vi "07-get-and_display_image.vi"() -> ()   [LabVIEW 2018, in "LV-0mq-Julia_roundtrip-lib.lvlib" / "LV2Julia_examples.lvlib"]
uses:
  LV2Julia_examples.lvlib
  LV2Julia_core/VIs/Server or client state.ctl
  LV2Julia_core/VIs/Commands.ctl
  c965f866-6df0-488f-ad0f-a92a8fae8aa7.vi
  f9264f0d-2c2d-4a22-a0da-9e005a3dfb77.vi
  c965f866-6df0-488f-ad0f-a92a8fae8aa7.vi/5d8143e1-f3ce-48d4-8562-fd4bfbe71124.vi
  f9264f0d-2c2d-4a22-a0da-9e005a3dfb77.vi/0c0e5131-77ab-4bc9-85bf-e376b45f74d3.vi
  c965f866-6df0-488f-ad0f-a92a8fae8aa7.vi/5d8143e1-f3ce-48d4-8562-fd4bfbe71124.vi/85423a51-09b0-429e-94d3-16956556064d.vi
  c965f866-6df0-488f-ad0f-a92a8fae8aa7.vi/5d8143e1-f3ce-48d4-8562-fd4bfbe71124.vi/311e7394-f85c-40bd-9389-6729e46b6738.vi
  c965f866-6df0-488f-ad0f-a92a8fae8aa7.vi/5d8143e1-f3ce-48d4-8562-fd4bfbe71124.vi/bf3cff3a-5cd2-4a77-8ee0-2dd55a1dd824.vi
  f9264f0d-2c2d-4a22-a0da-9e005a3dfb77.vi/0c0e5131-77ab-4bc9-85bf-e376b45f74d3.vi/ed46709f-38a3-410e-bde8-057d058233aa.vi
  f9264f0d-2c2d-4a22-a0da-9e005a3dfb77.vi/0c0e5131-77ab-4bc9-85bf-e376b45f74d3.vi/e79dc27b-6cb8-4aa6-a1cf-490a5ee80ef7.vi
  f9264f0d-2c2d-4a22-a0da-9e005a3dfb77.vi/0c0e5131-77ab-4bc9-85bf-e376b45f74d3.vi/d9315110-f036-4f78-83c6-5fac338d98fa.vi
  LV2Julia_core/VIs/check ID validity.vi
  LV2Julia_core/VIs/bindata_descr to JSON.vi
  LV2Julia_core/VIs/check cluster field names.vi
  LV2Julia_core/VIs/concat JSON.vi
  LV2Julia_core/VIs/build request.vi
  LV2Julia_core/VIs/Parse server response.vi
  LV2Julia_core/VIs/log jl exceptions.vi
  LV2Julia_core/VIs/jl-scripts path.vi
  LV2Julia_core/LV2Julia_core.lvlib
panel:
  out "img_type":string
  out "picture":picture
  in  "select image":u16(ring)
  out "short error info":string
  in  "next":bool
  out "current error":errorcluster
  out "final error":errorcluster
  in  "stop":bool
  out "ZMQ timeout":bool
  out "Julia script file path":path
  out "temporary script path":path
  out "Jl Server state":T1
  # "using TestImages, ImageMagick"
  # "If you don't see any received picture in this pane. check the scrollbars!"
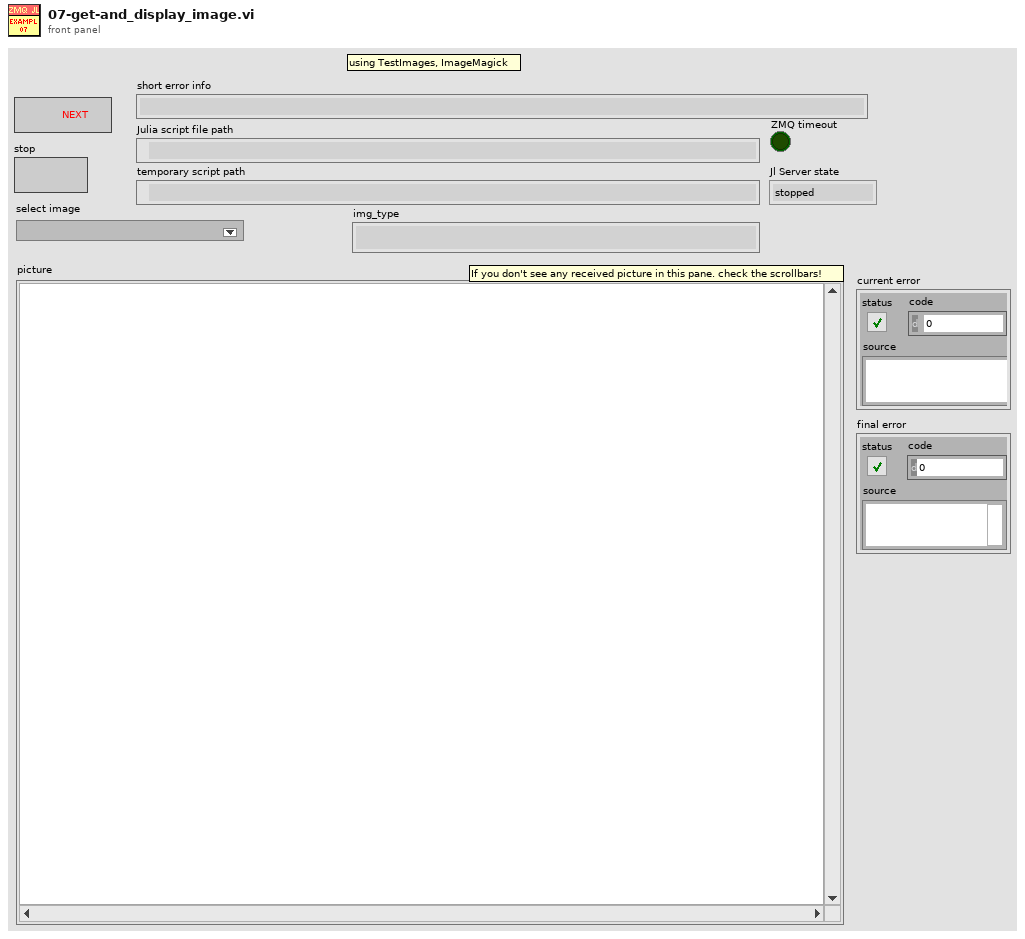
[diagram p1: front panel]
types:
  T1 = typedef "LV-0mq-Julia_roundtrip-lib.lvlib/LV2Julia_core.lvlib/Server or client state.ctl" = enum16{"stopped", "running", "unknown"}
  T2 = typedef "LV-0mq-Julia_roundtrip-lib.lvlib/LV2Julia_core.lvlib/Commands.ctl" = enum16{"Start Jl-server & Init LV-client", "Send request & Get response ", "Stop Jl-server & Cleanup LV-client", "Cleanup LV-client", "Start Jl-server", "Stop Jl-server", "Init LV-Client", "Cleanup LV-Client", "(not allowed)", "Set LV Client state", "Set Jl Server state", "set ZMQ timeout", "read ZMQ timeout", "read-out state"}
  T3 = typedef "LV-0mq-Julia_roundtrip-lib.lvlib/LV2Julia_core.lvlib/detailed error info.ctl" = cluster{"exception_or_info":string, "trace":T4[]}
  T4 = typedef "LV-0mq-Julia_roundtrip-lib.lvlib/LV2Julia_core.lvlib/StackFrame.ctl" = cluster{"frame_summary":string, "func":string, "linfo":string, "file":string, "line":i32, "pointer":u64, "from_c":bool, "inlined":bool}
  T5 = typedef "imagedata.ctl" = cluster{"image type":i32, "image depth":i32, "image":u8[], "mask":u8[], "colors":u32[], "Rectangle":cluster{"left":i16, "top":i16, "right":i16, "bottom":i16}}
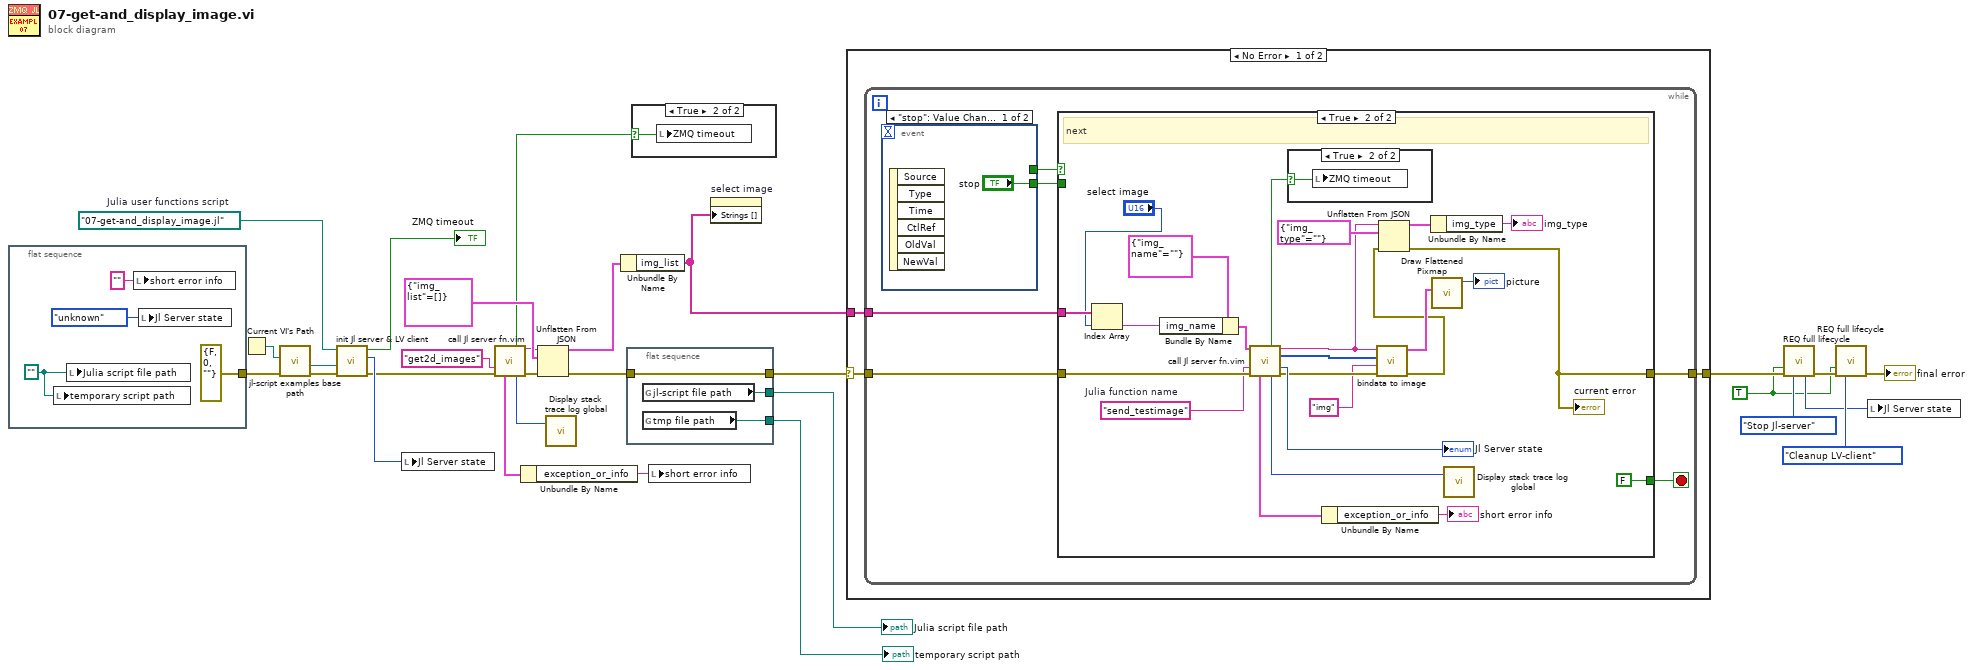
[diagram p0: block diagram]
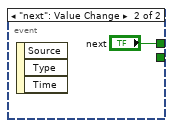
[diagram p3: hidden frame]
diagram:
  w8 = path "07-get-and_display_image.jl"  # Julia user functions script
  w20 = TRUE ("Force command")
  n1 = flat-sequence {
    tunnel: [errorcluster {"status"=FALSE, "code"=0, "source"=""} ("error in (no error)")] -> w2
    frame #0 {
      w31 = path ""
      n2 = local write "temporary script path"(w31) -> ()
      n3 = local write "Julia script file path"(w31) -> ()
      n4 = local write "short error info"("" ("short error info")) -> ()
      n5 = local write "Jl Server state"(Server_or_client_state."unknown" ("Jl Server state out")) -> ()
    }
  }
  n6 = Current VI's Path() -> (path=w4:path)
  n7 = call "jl-script examples base path.vi"("error in (no error)"=w2, "calling example VI path"=w4) -> ("error out"=w3:errorcluster, "jl-script-examples base path"=w1:path)  [unwired: 8 in]
  n8 = call "init Jl server & LV client.vi"("error in (no error)"=w3, "Base path (not a path)"=w1, "Julia user functions script"=w8) -> ("error out"=w5:errorcluster, "Jl Server state out"=w6:T1, "timeout?"=→"ZMQ timeout":bool)  [unwired: 6 in]
  n9 = local write "Jl Server state"(w6) -> ()
  n10 = call "call Jl server fn.vim"("fun2call"="get2d_images", "error in (no error)"=w5) -> ("timeout?"=w13:bool, "JSON received"=w15:string, "detailed error info"=w12:T3, "return code"=w10:u8, "error out"=w14:errorcluster)  [unwired: 7 in, 2 out]
  n11 = Unbundle By Name(w12) -> ("exception_or_info"=w11:string)
  n12 = Unflatten From JSON(JSON string=w15, type and defaults=cluster{"img_list":string[]} {"img_list"=[]} ("parsed response"), error in (no error)=w14) -> (value=w17:cluster{"img_list":string[]}, error out=w19:errorcluster)  [unwired: 4 in]
  n13 = call "Display stack trace log global.vi"("server return code"=w10) -> ()  [unwired: 3 in]
  n14 = Unbundle By Name(w17) -> ("img_list"=w9:string[])
  n15 = flat-sequence {
    tunnel: [w36] -> w24
    tunnel: w19 -> [w36]
    tunnel: [w35] -> w22
    tunnel: [w34] -> w23
    frame #0 {
      n16 = global read "jl-scripts path.vi" "jl-script file path"() -> (w35:path)
      n17 = global read "jl-scripts path.vi" "tmp file path"() -> (w34:path)
    }
  }
  n18 = case shown="True" w13 {
    selector: w13 -> [_ w37]
    frame False {
    }
    frame True {
      n19 = local write "ZMQ timeout"(w37) -> ()
    }
  }
  n20 = local write "short error info"(w11) -> ()
  n21 = property on="select image" class="Ring (strict)"("Strings []"=w9) -> ()  [unwired: 2 in, 2 out]
  n22 = case shown="No Error" w24 {
    selector: w24 -> [w39 w76]
    tunnel: [w40 w76] -> w29
    tunnel: w9 -> [w38 _]
    frame No Error {
      n23 = while {
        tunnel: w39 -> [w45]
        tunnel: [w46] -> w40
        tunnel: w38 -> [w41]
        stop <- w43 stop-if-true
        n24 = event shown="[0] \"stop\": Value Change" {
          selector: _ -> [_ _]
          dyn-events: _ -> [_ _]
          timeout: _ -> [_ _]
          tunnel: [_ "next"] -> w44
          tunnel: ["stop" _] -> w42
          event "stop": Value Change {
            n25 = event-data() -> ()  [unwired: 1 in, 6 out]
          }
          event "next": Value Change {
            n26 = event-data() -> ()  [unwired: 1 in, 3 out]
          }
        }
        n27 = case shown="True" w44 {
          tunnel: [w50 w52] -> w46
          tunnel: w45 -> [w50 w73]
          tunnel: [w49 FALSE ("stop this VI only")] -> w43
          tunnel: w42 -> [w49 _]
          tunnel: w41 -> [_ w64]
          frame False {
            # "stop"
          }
          frame True {
            w72 = "send_testimage"  # Julia function name
            # "next"
            n28 = Index Array(array=w64, index="select image") -> (element=w65:string)
            n29 = Bundle By Name(cluster=cluster{"img_name":string} {"img_name"=""} ("parsed response"), "img_name"=w65) -> (w62:cluster{"img_name":string})
            n30 = call "call Jl server fn.vim"("Arguments 1"=w62, "fun2call"=w72, "error in (no error)"=w73) -> ("timeout?"=w70:bool, "JSON received"=w51:string, "binary data received"=w58:u8[], "Jl Server state out"=→"Jl Server state":T1, "detailed error info"=w68:T3, "return code"=w69:u8, "error out"=w59:errorcluster)  [unwired: 6 in]
            n31 = case shown="True" w70 {
              selector: w70 -> [_ w75]
              frame False {
              }
              frame True {
                n32 = local write "ZMQ timeout"(w75) -> ()
              }
            }
            n33 = Unbundle By Name(w68) -> ("exception_or_info"=→"short error info":string)
            n34 = call "bindata to image.vi"("error in (no error)"=w59, "name"="img", "binary data in"=w58, "JSON in"=w51) -> ("error out"=w53:errorcluster, "img out"=w60:T5)  [unwired: 6 in]
            n35 = Unflatten From JSON(JSON string=w51, type and defaults=cluster{"img_type":string} {"img_type"=""}, error in (no error)=w53) -> (value=w55:cluster{"img_type":string}, error out=w52:errorcluster)  [unwired: 4 in]
            "current error" <- w52
            n36 = Unbundle By Name(w55) -> ("img_type"=→"img_type":string)
            n37 = call <vilib>:"Draw Flattened Pixmap.vi"("image data"=w60) -> ("new picture"=→"picture":picture)  [unwired: 8 in]
            n38 = call "Display stack trace log global.vi"("server return code"=w69) -> ()  [unwired: 3 in]
          }
        }
      }
    }
    frame Error {
    }
  }
  n39 = call "REQ full lifecycle.vi"("Force command"=w20, "error in"=w29, "command"=Commands."Stop Jl-server") -> ("Jl Server state out"=w21:T1, "error out"=w27:errorcluster)  [unwired: 6 in, 5 out]
  n40 = call "REQ full lifecycle.vi"("Force command"=w20, "error in"=w27, "command"=Commands."Cleanup LV-client") -> ("error out"=→"final error":errorcluster)  [unwired: 6 in, 6 out]
  n41 = local write "Jl Server state"(w21) -> ()
  "temporary script path" <- w23
  "Julia script file path" <- w22
